vi "Soft Stop Demo.vi"() -> ()   [LabVIEW 2012]
panel:
  in  "pause":bool
  out "Motor Out":dbl
  out "At Hi":bool
  out "At Lo":bool
  in  "Disable Softstops":bool
  in  "Disable Motor":bool
  in  "Motor In":dbl(slide)=0.04 scale=-1.0..1.0
  in  "Lo Limit":dbl=-10.0
  in  "Hi Limit":dbl=35.0
  out "sense":dbl
  in  "reset":bool
  in  "correlation":bool=TRUE
  out "Waveform Chart":dbl(graph)
  in  "Margin":dbl=1.0
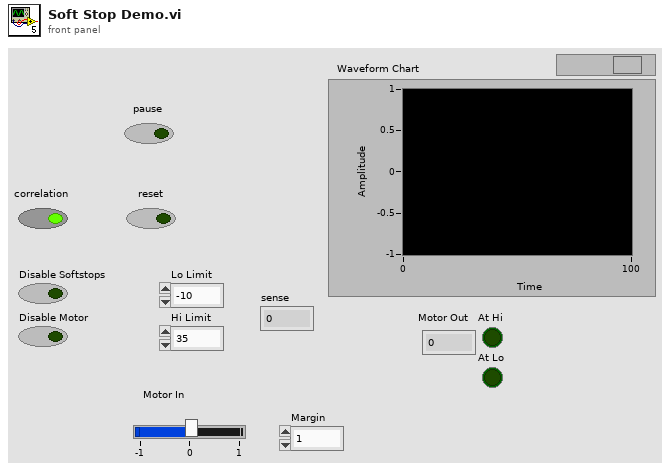
[diagram p1: front panel]
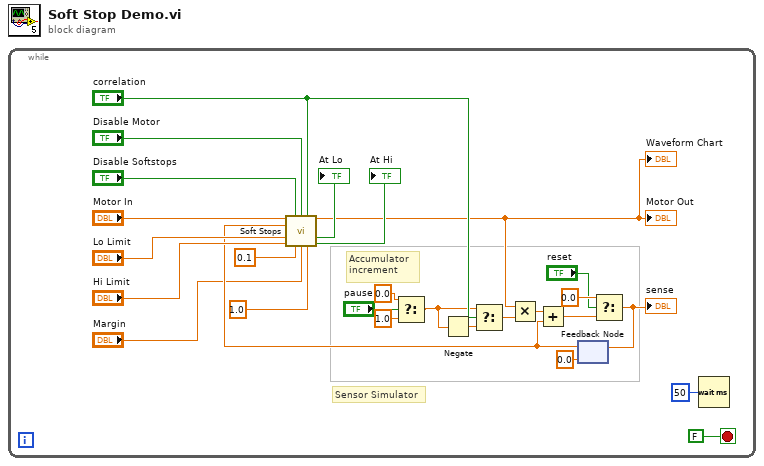
[diagram p0: block diagram]
diagram:
  n1 = while {
    stop <- FALSE stop-if-true
    # "Sensor Simulator"
    # "Accumulator\nincrement"
    n2 = Select(t=0.0, s="pause", f=1.0) -> (s? t:f=w4:dbl)
    n3 = Negate(x=w4) -> (-x=w15:dbl)
    n4 = Select(t=w4, s="correlation", f=w15) -> (s? t:f=w16:dbl)
    n5 = feedback #1(0.0 ("t")) -> (w10:dbl)
    n6 = call "Soft Stops.vi"("Motor In"="Motor In", "Disable Softstops"="Disable Softstops", "Disable Motor"="Disable Motor", "correlation"="correlation", "Sense"=w10, "Lo Limit"="Lo Limit", "Hi Limit"="Hi Limit", "Speed near Limit"=0.1, "Margin"="Margin", "Motor Coerce"=1.0) -> ("Motor Out"=w6:dbl, "At Lo"=→"At Lo":bool, "At Hi"=→"At Hi":bool)  [unwired: 3 in]
    "Motor Out" <- w6
    "Waveform Chart" <- w6
    n7 = Multiply(x=w6, y=w16) -> (x*y=w20:dbl)
    n8 = Add(x=w20, y=w10) -> (x+y=w19:dbl)
    n9 = Select(t=0.0, s="reset", f=w19) -> (s? t:f=w14:dbl)
    "sense" <- w14
    n10 = feedback-in #1(w14) -> ()
    n11 = Wait (ms)(milliseconds to wait=u32 50) -> ()  [unwired: 1 out]
  }
